vi "Add documentation to vis.vi"() -> ()   [LabVIEW 2010]
doc: "This .vi helps one add documentation to a list of .vis"
panel:
  in  "Numeric":i32
  out "file":string
  in  "Done":bool
  in  "Documentation":string
  in  "Files to Document (paste data here)":string[](array[string])
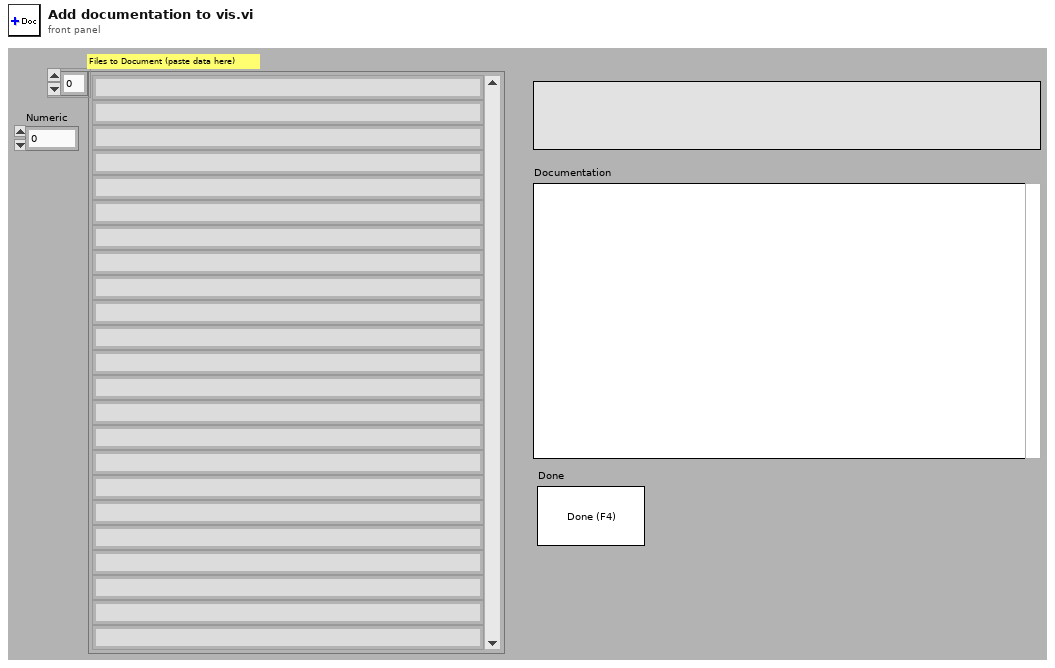
[diagram p1: front panel]
types:
  T1 = enum32{"Invalid", "Standard", "Closed", "Hidden", "Minimized", "Maximized"}
  T2 = typedef "LVRectTypeDef.ctl" = cluster{"left":i16, "top":i16, "right":i16, "bottom":i16}
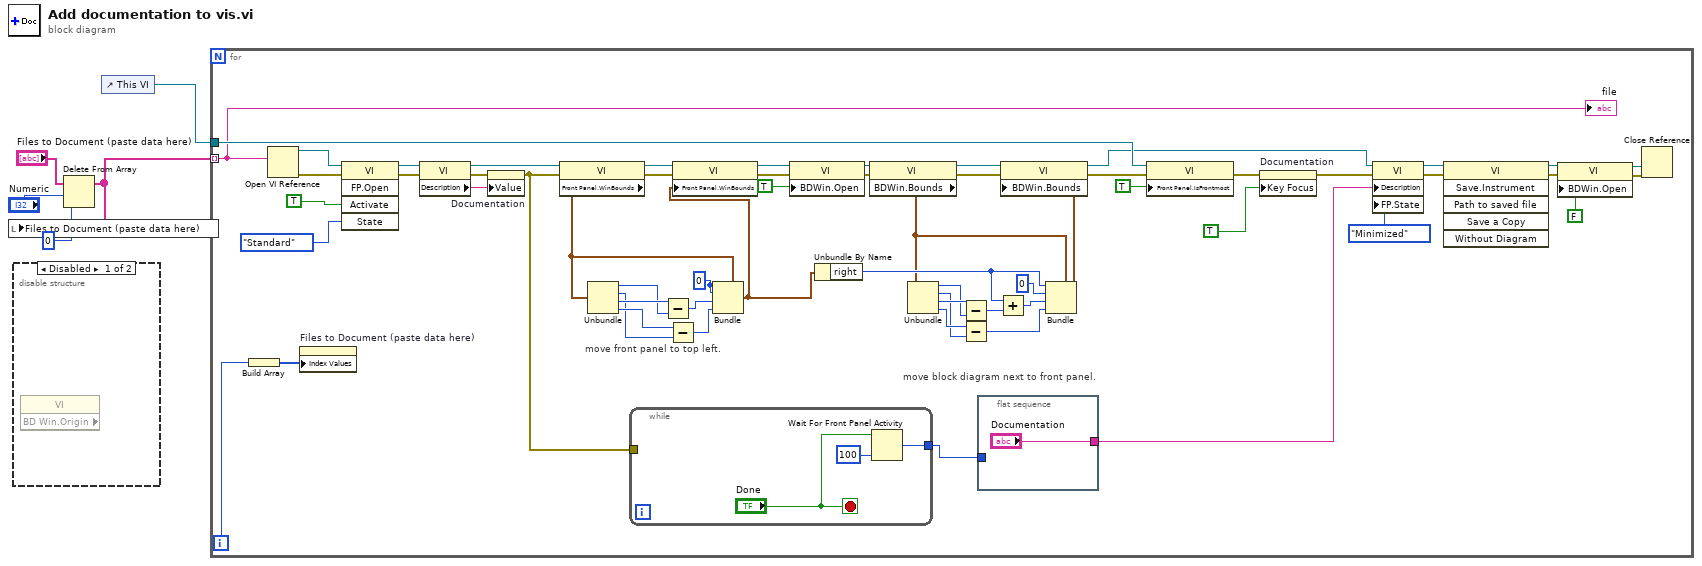
[diagram p0: block diagram]
diagram:
  n1 = disable-structure shown="Disabled" {
    frame Disabled {
      n2 = property class="VI" props=["BD Win.Origin"]() -> ()  [unwired: 2 in, 3 out]
    }
    frame Enabled {
    }
  }
  n3 = Delete From Array(array="Files to Document (paste data here)", length="Numeric", index=0) -> (array with subset deleted=w2:string[])  [unwired: 1 out]
  n4 = local write "Files to Document (paste data here)"(w2) -> ()
  n5 = control-ref of="This VI"() -> (w5:refnum<vi>)
  n6 = for {
    tunnel: w2 -> [w51] mode=indexing
    tunnel: w5 -> [w54]
    i -> [w9]
    w41 = i16 0 ("left")
    # "move block diagram next to front panel."
    # "move front panel to top left."
    n7 = Build Array(w9) -> (w8:i32[])
    n8 = Open VI Reference(vi path=w51) -> (vi reference=w63:refnum<vi>, error out=w64:errorcluster)  [unwired: 1 in, 4 out]
    n9 = property on="Files to Document (paste data here)" class="Arr (strict)"("Index Values"=w8) -> ()  [unwired: 2 in, 2 out]
    n10 = invoke class="VI" method="FP.Open"(reference=w63, error in=w64, "Activate"=TRUE ("Activate?"), "State"=T1."Standard") -> (reference out=w12:refnum<vi>, error out=w11:errorcluster)  [unwired: 1 in, 3 out]
    n11 = property class="VI"(reference=w12, error in=w11) -> (reference out=w13:refnum<vi>, error out=w53:errorcluster, "Description"=w52:string)
    n12 = property on="Documentation" class="Str"(error in=w53, "Value"=w52) -> (error out=w10:errorcluster)  [unwired: 1 in, 1 out]
    n13 = property class="VI"(reference=w13, error in=w10) -> (reference out=w40:refnum<vi>, error out=w39:errorcluster, "Front Panel.WinBounds"=w7:T2)
    n14 = Unbundle(w7) -> ("left"=w44:i16, "top"=w45:i16, "right"=w47:i16, "bottom"=w46:i16)
    n15 = while {
      tunnel: [w66] -> w48
      tunnel: w10 -> [_]
      stop <- "Done" stop-if-true
      n16 = Wait For Front Panel Activity(1:100 ("timeout ms (-1 never timeout)"), 3:"Done") -> (0:w66:u32)  [unwired: 1 out]
    }
    n17 = Subtract(x=w47, y=w44) -> (x-y=w42:i16)
    n18 = Subtract(x=w46, y=w45) -> (x-y=w43:i16)
    n19 = Bundle(cluster=w7, "left"=w41, "top"=w41, "right"=w42, "bottom"=w43) -> (w29:T2)
    n20 = property class="VI"(reference=w40, error in=w39, "Front Panel.WinBounds"=w29) -> (reference out=w38:refnum<vi>, error out=w37:errorcluster)
    n21 = property class="VI"(reference=w38, error in=w37, "BDWin.Open"=TRUE ("Block Diagram Window:Open")) -> (reference out=w35:refnum<vi>, error out=w34:errorcluster)
    n22 = Unbundle By Name(w29) -> ("right"=w25:i16)
    n23 = property class="VI"(reference=w35, error in=w34) -> (reference out=w33:refnum<vi>, error out=w32:errorcluster, "BDWin.Bounds"=w6:T2)
    n24 = Unbundle(w6) -> ("left"=w27:i16, "top"=w22:i16, "right"=w28:i16, "bottom"=w23:i16)
    n25 = Subtract(x=w28, y=w27) -> (x-y=w26:i16)
    n26 = Subtract(x=w23, y=w22) -> (x-y=w21:i16)
    n27 = flat-sequence {
      tunnel: ["Documentation"] -> w59
      tunnel: w48 -> [_]
      frame #0 {
      }
    }
    n28 = Add(x=w25, y=w26) -> (x+y=w24:i16)
    n29 = Bundle(cluster=w6, "left"=w25, "top"=i16 0 ("left"), "right"=w24, "bottom"=w21) -> (w31:T2)
    n30 = property class="VI"(reference=w33, error in=w32, "BDWin.Bounds"=w31) -> (reference out=w15:refnum<vi>, error out=w14:errorcluster)
    n31 = property class="VI"(reference=w54, error in=w14, "Front Panel.IsFrontmost"=TRUE ("Front Panel Window:Is Frontmost")) -> (error out=w56:errorcluster)  [unwired: 1 out]
    n32 = property on="Documentation" class="Str"(error in=w56, "Key Focus"=TRUE) -> (error out=w60:errorcluster)  [unwired: 1 in, 1 out]
    n33 = property class="VI"(reference=w15, error in=w60, "Description"=w59, "FP.State"=T1."Minimized" ("Front Panel Window:State")) -> (reference out=w50:refnum<vi>, error out=w49:errorcluster)
    n34 = invoke class="VI" method="Save.Instrument"(reference=w50, error in=w49) -> (reference out=w20:refnum<vi>, error out=w19:errorcluster)  [unwired: 4 in, 4 out]
    n35 = property class="VI"(reference=w20, error in=w19, "BDWin.Open"=FALSE ("Key Focus")) -> (reference out=w18:refnum<vi>, error out=w17:errorcluster)
    n36 = Close Reference(reference=w18, error in (no error)=w17) -> ()  [unwired: 1 out]
    "file" <- w51
  }
